vi "Configure Marker Search.vi"(7 "Marker Search":T1(ring), 8 "error in (no error)":errorcluster, 9 "Target Value":dbl, 10 "Marker Number":u8=1, 11 "VNA-ENA in":refnum<class "VNA-ENA.lvclass">) -> (0 "error out":errorcluster, 3 "VNA-ENA out":refnum<class "VNA-ENA.lvclass">)   [LabVIEW 2020, in "VNA-ENA.lvclass"]
doc: "Configures and excecutes a marker search.\nThe marker is on the active trace."
uses:
  VNA-ENA.lvclass
  C:/Sandbox/Git_Sandbox/WiSpry Test Framework source code (LV20)/WiSpry Test Framework/Instruments/Instrument.lvclass
  Instrument.lvclass/Instrument.ctl
  Instrument.lvclass
  <instrlib>/Agilent ENA Series/Agilent ENA Series.lvlib
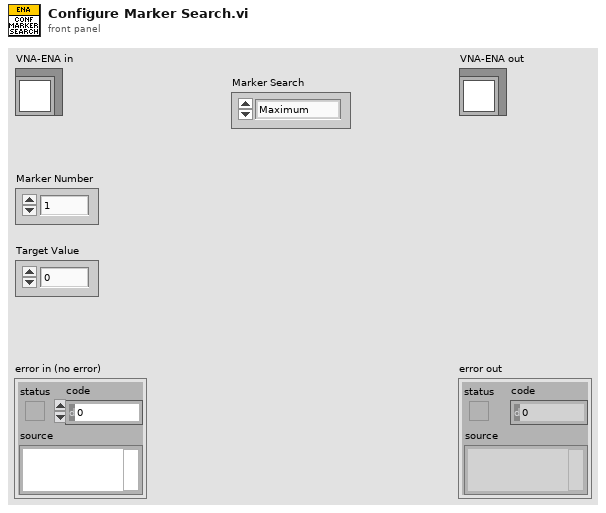
[diagram p1: front panel]
types:
  T1 = enum16{"Maximum", "Minimum", "Right Peak", "Left Peak", "Negative Peak", "Taget Value", "Left Taget Value", "Rigth Target Value"}
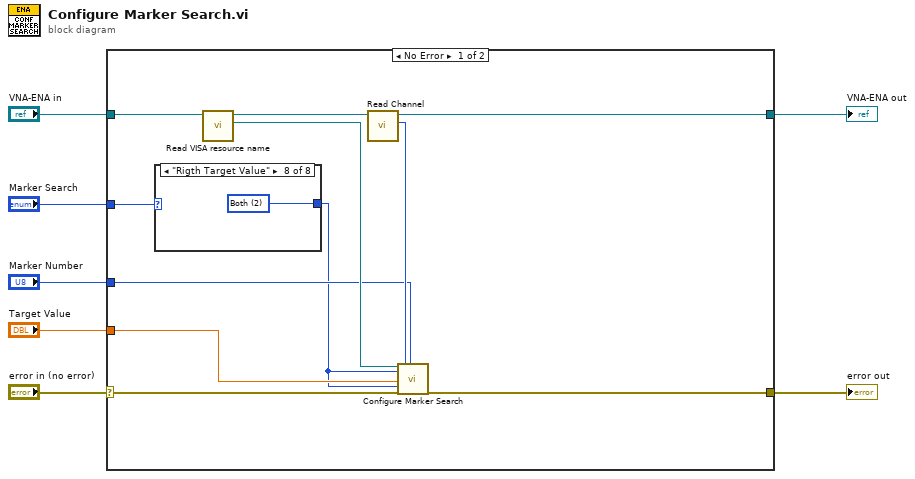
[diagram p0: block diagram]
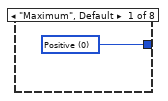
[diagram p2: hidden frame]
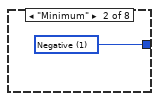
[diagram p3: hidden frame]
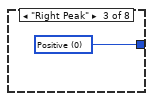
[diagram p4: hidden frame]
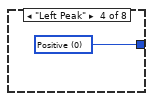
[diagram p5: hidden frame]
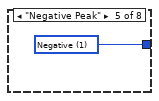
[diagram p6: hidden frame]
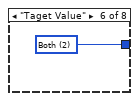
[diagram p7: hidden frame]
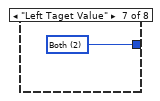
[diagram p8: hidden frame]
diagram:
  n1 = case shown="No Error" "error in (no error)" {
    selector: "error in (no error)" -> [w17 w28]
    tunnel: [w16 w28] -> w4
    tunnel: [w14 w27] -> w5
    tunnel: "VNA-ENA in" -> [w18 w27]
    tunnel: "Target Value" -> [w11 _]
    tunnel: "Marker Search" -> [w10 _]
    tunnel: "Marker Number" -> [w9 _]
    frame No Error {
      n2 = case shown="\"Rigth Target Value\"" w10 {
        tunnel: [w19 w20 w21 w22 w23 w24 w25 w26] -> w8
        frame "Maximum", Default {
          w19 = u16 0 items=["Positive", "Negative", "Both"] ("Peak Polarity (0: Positive)")
        }
        frame "Minimum" {
          w20 = u16 1 items=["Positive", "Negative", "Both"] ("Peak Polarity (0: Positive)")
        }
        frame "Right Peak" {
          w21 = u16 0 items=["Positive", "Negative", "Both"] ("Peak Polarity (0: Positive)")
        }
        frame "Left Peak" {
          w22 = u16 0 items=["Positive", "Negative", "Both"] ("Peak Polarity (0: Positive)")
        }
        frame "Negative Peak" {
          w23 = u16 1 items=["Positive", "Negative", "Both"] ("Peak Polarity (0: Positive)")
        }
        frame "Taget Value" {
          w24 = u16 2 items=["Positive", "Negative", "Both"] ("Peak Polarity (0: Positive)")
        }
        frame "Left Taget Value" {
          w25 = u16 2 items=["Positive", "Negative", "Both"] ("Peak Polarity (0: Positive)")
        }
        frame "Rigth Target Value" {
          w26 = u16 2 items=["Positive", "Negative", "Both"] ("Peak Polarity (0: Positive)")
        }
      }
      n3 = call "Read VISA resource name.vi"("Instrument in"=w18) -> ("VISA resource name"=w12:refnum<visa-resource-name>, "Instrument out"=w15:refnum<class "VNA-ENA.lvclass">)  [unwired: 9 in]
      n4 = call-dynamic "Read Channel.vi"("Vector Network Analyzer in"=w15) -> ("Channel"=w13:i32, "Vector Network Analyzer out"=w14:refnum<class "VNA-ENA.lvclass">)  [unwired: 9 in]
      n5 = call <instrlib>:"Configure Marker Search.vi"("VISA resource name"=w12, "Peak Polarity (0: Positive)"=w8, "Target Value (0.0)"=w11, "Target Polarity (0: Positive)"=w8, "error in (no error)"=w17, "Channel (1)"=w13, "Marker (1)"=w9) -> ("error out"=w16:errorcluster)  [unwired: 11 in, 1 out]
    }
    frame Error {
    }
  }
  "error out" <- w4
  "VNA-ENA out" <- w5
